vi "write da x.vi"(8 "error in (no error)":errorcluster, 10 "value":u16, 11 "x":u16) -> (0 "error out":errorcluster)   [LabVIEW 2015, in "SCANalone4x64.lvlib"]
doc: "__declspec(dllimport) void __stdcall write_da_x(unsigned short x, unsigned short value);"
uses:
  <userlib>/SCANalone4x64/SCANalone4x64.lvlib
  <userlib>/SCANalone4x64/SCANalone4x64.dll
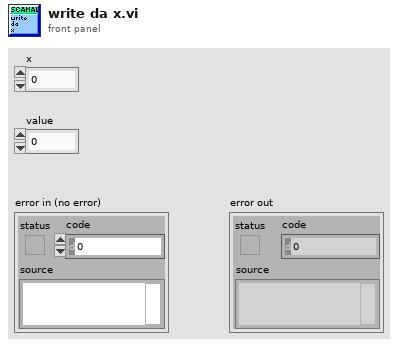
[diagram p1: front panel]
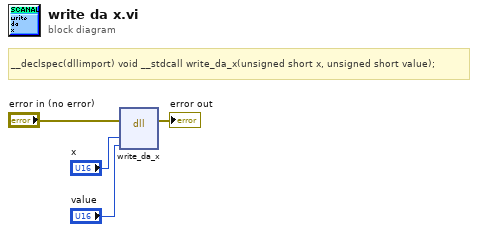
[diagram p0: block diagram]
diagram:
  # "__declspec(dllimport) void __stdcall write_da_x(unsigned short x, unsigned short value);"
  n1 = dll-call lib="C:/Program Files/National Instruments/LabVIEW 2015/user.lib/SCANalone4x64/SCANalone4x64.*" fn="write_da_x"(error in="error in (no error)", "x"="x", "value"="value") -> (error out=→"error out":errorcluster)  [unwired: 5 in, 1 out]
